vi "set single axis Field Module.vi"(0 "Field Device Select":string(combo)="Elsa Magnet mT", 1 "Field sub select":string(combo)="50mApV", 5 "error in (no error)":errorcluster, 6 "Power dbm":dbl=-135.0 format="%#_13g", 7 "Init":bool, 8 "Field Target mT or dBm":dbl format="%#_13g", 9 "Exec":bool, 10 "Field Rate mT per sec":dbl=0.1 format="%#_13g", 11 "final":bool) -> (19 "error out":errorcluster)   [LabVIEW 2024]
panel:
  out "Voltage controlled Field mT 2":dbl
  in  "E8257 VISA":refnum<visa-resource-name>="GPIB0::19::INSTR"
  out "Current FIeld mT":dbl
  out "Voltage controlled Field mT":dbl
  # "1mT =?V"
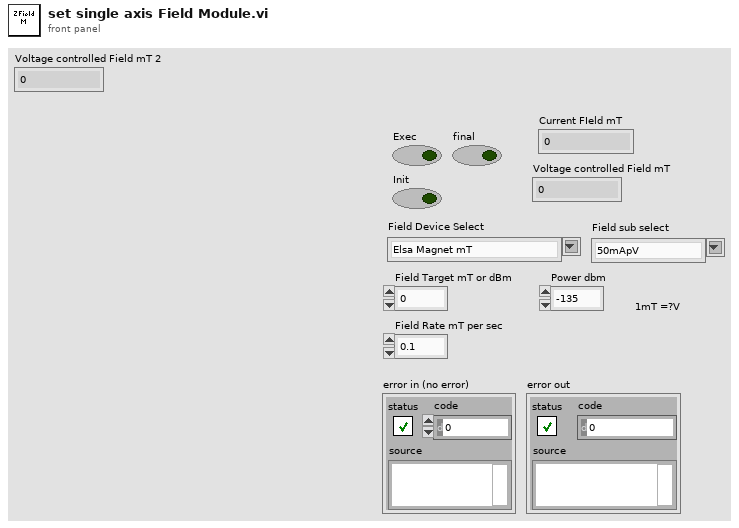
[diagram p1: front panel]
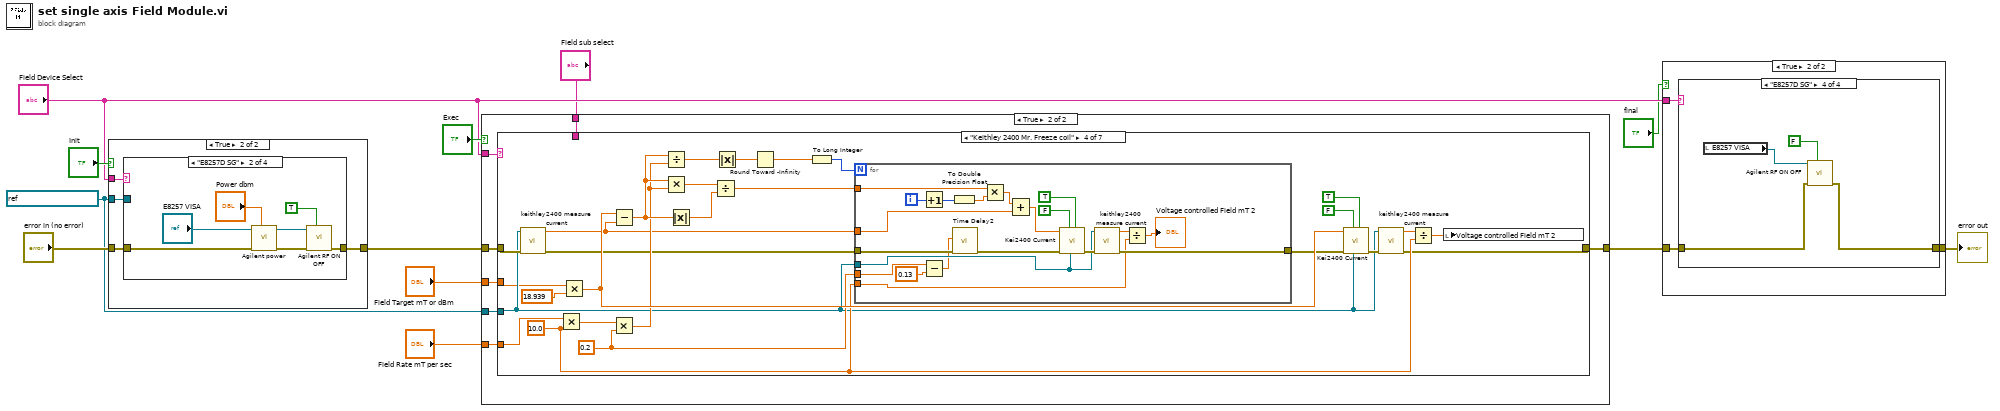
[diagram p0: block diagram]
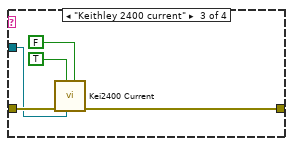
[diagram p8: hidden frame]
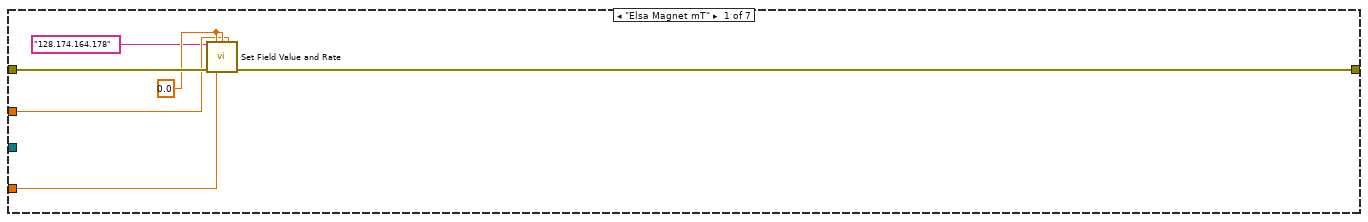
[diagram p11: hidden frame]
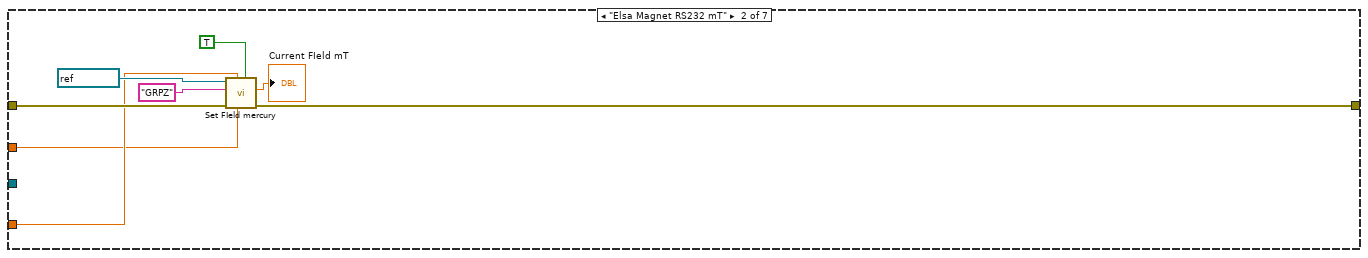
[diagram p12: hidden frame]
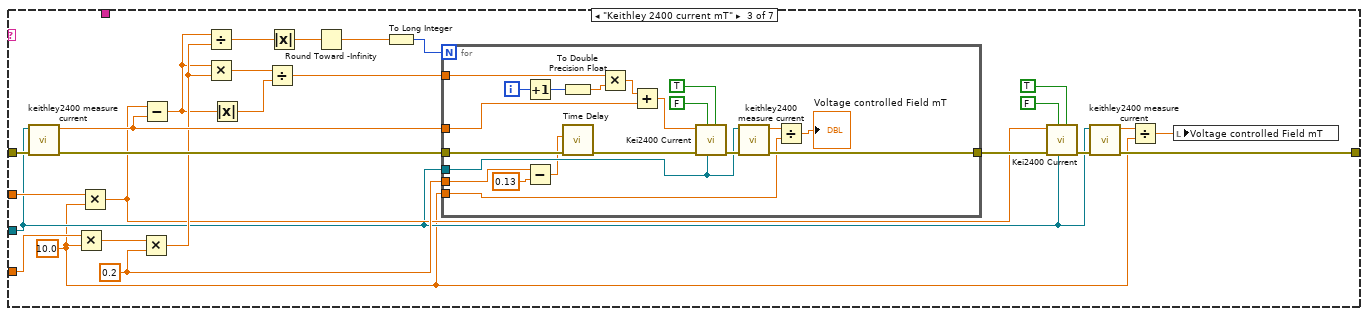
[diagram p13: hidden frame]
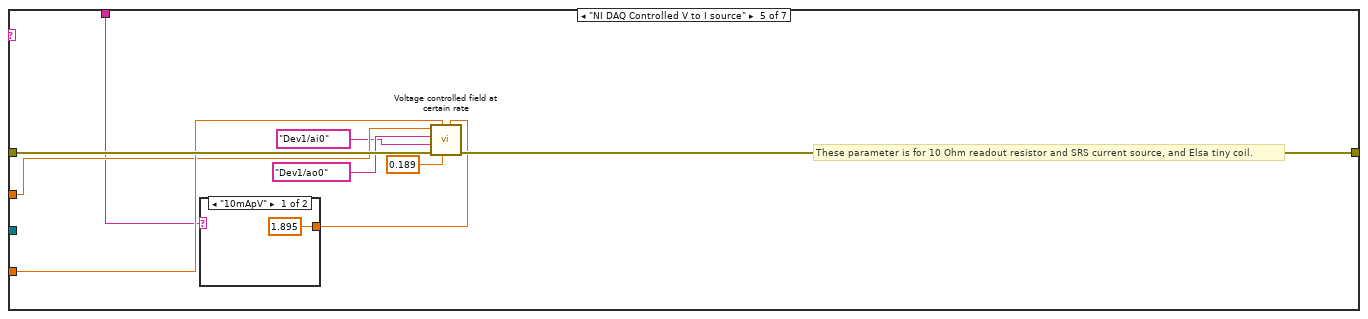
[diagram p14: hidden frame]
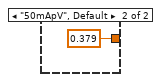
[diagram p15: hidden frame]
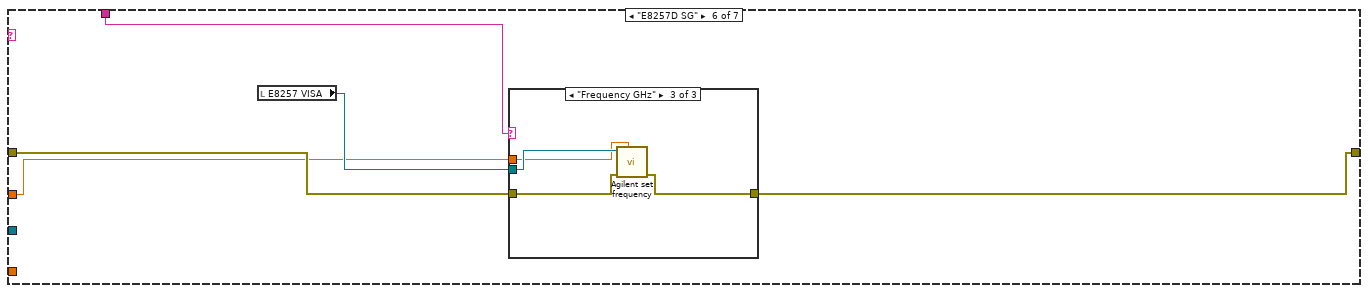
[diagram p16: hidden frame]
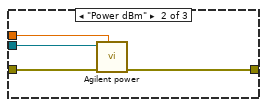
[diagram p18: hidden frame]
diagram:
  w2 = refnum<visa-resource-name> "GPIB0::26::INSTR" ("VISA resource name")
  n1 = case shown="True" "Init" {
    tunnel: "error in (no error)" -> [w13 w17]
    tunnel: [w13 w16] -> w7
    tunnel: "Field Device Select" -> [_ w15]
    tunnel: w2 -> [_ w14]
    frame False {
    }
    frame True {
      n2 = case shown="\"E8257D SG\"" w15 {
        tunnel: w17 -> [w18 w25 w28 w31]
        tunnel: [w18 w19 w27 w31] -> w16
        tunnel: w14 -> [_ _ w26 _]
        frame "Elsa Magnet" {
        }
        frame "E8257D SG" {
          n3 = call "Agilent power.vi"("Power dbm"="Power dbm", "error in (no error)"=w25, "VISA resource name"="E8257 VISA") -> ("error out"=w21:errorcluster, "VISA resource name out"=w22:refnum<visa-resource-name>)  [unwired: 7 in]
          n4 = call "Agilent RF ON OFF.vi"("Output Enable"=TRUE, "error in (no error)"=w21, "VISA resource name"=w22) -> ("error out"=w19:errorcluster)  [unwired: 7 in, 1 out]
        }
        frame "Keithley 2400 current" {
          n5 = call "Kei2400 Current.vi"("Exec"=FALSE, "VISA resource name"=w26, "Init"=TRUE, "error in (no error)"=w28) -> ("error out"=w27:errorcluster)  [unwired: 7 in]
        }
        frame "None", Default {
        }
      }
    }
  }
  n6 = case shown="True" "Exec" {
    tunnel: w7 -> [w32 w39]
    tunnel: [w32 w34] -> w5
    tunnel: "Field Target mT or dBm" -> [_ w38]
    tunnel: "Field Rate mT per sec" -> [_ w37]
    tunnel: "Field Device Select" -> [_ w36]
    tunnel: w2 -> [_ w35]
    tunnel: "Field sub select" -> [_ w33]
    frame False {
    }
    frame True {
      n7 = case shown="\"Keithley 2400 Mr. Freeze coil\"" w36 {
        tunnel: w39 -> [w45 w53 w78 w103 w155 w161 w172]
        tunnel: w38 -> [w42 w48 w79 w101 w153 w159 _]
        tunnel: w37 -> [w41 w49 w77 w104 w154 _ _]
        tunnel: w35 -> [_ _ w57 w102 _ _ _]
        tunnel: [w44 w50 w58 w105 w150 w160 w172] -> w34
        tunnel: w33 -> [_ _ _ _ w147 w158 _]
        frame "Elsa Magnet mT" {
          w43 = 0.0 ("Target Field X kG")
          n8 = call "Set Field Value and Rate.vi"("IP Address"="128.174.164.178", "Target Field X mT"=w43, "Target Field Y mT"=w43, "Target Field Z mT"=w42, "error in (no error)"=w45, "Ramp Rate mT per s"=w41) -> ("error out"=w44:errorcluster)  [unwired: 9 in]
        }
        frame "Elsa Magnet RS232 mT" {
          n9 = call "Set FIeld mercury.vi"("wait for hold"=TRUE, "FIeld mT"=w48, "FIeld mT  per sec"=w49, "error in (no error)"=w53, "Device on PSU"="GRPZ", "VISA resource name"=refnum<visa-resource-name> "COM1") -> ("error out"=w50:errorcluster, "Current FIeld mT"=→"Current FIeld mT":dbl)  [unwired: 3 in, 1 out]
        }
        frame "Keithley 2400 current mT" {
          w72 = 0.2 ("y")
          w54 = 10.0 ("y")
          n10 = call "keithley2400 measure current.vi"("error in (no error)"=w78, "VISA resource name"=w57) -> ("error out"=w75:errorcluster, "Current mA"=w73:dbl)  [unwired: 8 in]
          n11 = Multiply(x=w77, y=w54) -> (x*y=w76:dbl)
          n12 = Multiply(x=w79, y=w54) -> (x*y=w62:dbl)
          n13 = Multiply(x=w76, y=w72) -> (x*y=w71:dbl)
          n14 = Subtract(x=w62, y=w73) -> (x-y=w69:dbl)
          n15 = Divide(x=w69, y=w71) -> (x/y=w74:dbl)
          n16 = Multiply(x=w69, y=w71) -> (x*y=w70:dbl)
          n17 = Absolute Value(x=w69) -> (abs(x)=w68:dbl)
          n18 = Divide(x=w70, y=w68) -> (x/y=w67:dbl)
          n19 = Absolute Value(x=w74) -> (abs(x)=w66:dbl)
          n20 = Round Toward -Infinity(1:w66) -> (0:w65:dbl)
          n21 = To Long Integer(number=w65) -> (32bit integer=w64:i32)
          n22 = for {
            N: w64 -> [_]
            tunnel: w57 -> [w88]
            tunnel: w75 -> [w92]
            tunnel: [w86] -> w63
            tunnel: w73 -> [w93]
            tunnel: w72 -> [w85]
            tunnel: w67 -> [w90]
            tunnel: w54 -> [w80]
            i -> [w97]
            n23 = Increment(x=w97) -> (x+1=w96:i32)
            n24 = Subtract(x=w85, y=0.13) -> (x-y=w83:dbl)
            n25 = To Double Precision Float(number=w96) -> (double precision float=w95:dbl)
            n26 = call "Time Delay"("error in (no error)"=w92, "Delay Time (s)"=w83) -> ("error out"=w87:errorcluster)  [unwired: 9 in]
            n27 = Multiply(x=w90, y=w95) -> (x*y=w94:dbl)
            n28 = Add(x=w94, y=w93) -> (x+y=w91:dbl)
            n29 = call "Kei2400 Current.vi"("Exec"=TRUE, "VISA resource name"=w88, "Init"=FALSE, "error in (no error)"=w87, "Current mA"=w91) -> ("error out"=w89:errorcluster)  [unwired: 6 in]
            n30 = call "keithley2400 measure current.vi"("error in (no error)"=w89, "VISA resource name"=w88) -> ("error out"=w86:errorcluster, "Current mA"=w81:dbl)  [unwired: 8 in]
            n31 = Divide(x=w81, y=w80) -> (x/y=→"Voltage controlled Field mT":dbl)
          }
          n32 = call "Kei2400 Current.vi"("Exec"=TRUE, "VISA resource name"=w57, "Init"=FALSE, "error in (no error)"=w63, "Current mA"=w62) -> ("error out"=w59:errorcluster)  [unwired: 6 in]
          n33 = call "keithley2400 measure current.vi"("error in (no error)"=w59, "VISA resource name"=w57) -> ("error out"=w58:errorcluster, "Current mA"=w55:dbl)  [unwired: 8 in]
          n34 = Divide(x=w55, y=w54) -> (x/y=w56:dbl)
          n35 = local write "Voltage controlled Field mT"(w56) -> ()
        }
        frame "Keithley 2400 Mr. Freeze coil" {
          w108 = 0.2 ("y")
          w109 = 10.0 ("y")
          n36 = call "keithley2400 measure current.vi"("error in (no error)"=w103, "VISA resource name"=w102) -> ("error out"=w111:errorcluster, "Current mA"=w113:dbl)  [unwired: 8 in]
          n37 = Multiply(x=w104, y=w109) -> (x*y=w110:dbl)
          n38 = Multiply(x=w101, y=18.939) -> (x*y=w123:dbl)
          n39 = Multiply(x=w110, y=w108) -> (x*y=w114:dbl)
          n40 = Subtract(x=w123, y=w113) -> (x-y=w116:dbl)
          n41 = Divide(x=w116, y=w114) -> (x/y=w112:dbl)
          n42 = Multiply(x=w116, y=w114) -> (x*y=w115:dbl)
          n43 = Absolute Value(x=w116) -> (abs(x)=w117:dbl)
          n44 = Divide(x=w115, y=w117) -> (x/y=w118:dbl)
          n45 = Absolute Value(x=w112) -> (abs(x)=w119:dbl)
          n46 = Round Toward -Infinity(1:w119) -> (0:w120:dbl)
          n47 = To Long Integer(number=w120) -> (32bit integer=w121:i32)
          n48 = for {
            N: w121 -> [_]
            tunnel: w102 -> [w135]
            tunnel: w111 -> [w139]
            tunnel: [w133] -> w122
            tunnel: w113 -> [w140]
            tunnel: w108 -> [w132]
            tunnel: w118 -> [w137]
            tunnel: w109 -> [w127]
            i -> [w144]
            n49 = Increment(x=w144) -> (x+1=w143:i32)
            n50 = Subtract(x=w132, y=0.13) -> (x-y=w130:dbl)
            n51 = To Double Precision Float(number=w143) -> (double precision float=w142:dbl)
            n52 = call "Time Delay2"("error in (no error)"=w139, "Delay Time (s)"=w130) -> ("error out"=w134:errorcluster)  [unwired: 9 in]
            n53 = Multiply(x=w137, y=w142) -> (x*y=w141:dbl)
            n54 = Add(x=w141, y=w140) -> (x+y=w138:dbl)
            n55 = call "Kei2400 Current.vi"("Exec"=TRUE, "VISA resource name"=w135, "Init"=FALSE, "error in (no error)"=w134, "Current mA"=w138) -> ("error out"=w136:errorcluster)  [unwired: 6 in]
            n56 = call "keithley2400 measure current.vi"("error in (no error)"=w136, "VISA resource name"=w135) -> ("error out"=w133:errorcluster, "Current mA"=w128:dbl)  [unwired: 8 in]
            n57 = Divide(x=w128, y=w127) -> (x/y=→"Voltage controlled Field mT 2":dbl)
          }
          n58 = call "Kei2400 Current.vi"("Exec"=TRUE, "VISA resource name"=w102, "Init"=FALSE, "error in (no error)"=w122, "Current mA"=w123) -> ("error out"=w124:errorcluster)  [unwired: 6 in]
          n59 = call "keithley2400 measure current.vi"("error in (no error)"=w124, "VISA resource name"=w102) -> ("error out"=w105:errorcluster, "Current mA"=w126:dbl)  [unwired: 8 in]
          n60 = Divide(x=w126, y=w109) -> (x/y=w125:dbl)
          n61 = local write "Voltage controlled Field mT 2"(w125) -> ()
        }
        frame "NI DAQ Controlled V to I source" {
          # "These parameter is for 10 Ohm readout resistor and SRS current source, and Elsa tiny coil."
          n62 = case shown="\"10mApV\"" w147 {
            tunnel: [1.895 ("output voltage per mT") 0.379 ("output voltage per mT")] -> w149
            frame "10mApV" {
            }
            frame "50mApV", Default {
            }
          }
          n63 = call "Voltage controlled field at certain rate.vi"("action voltage per mT"=w149, "Readout voltage per mT"=0.189 ("intput voltage per mT"), "Rate mT per sec"=w154, "error in (no error)"=w155, "Voltage read channel"=tag "Dev1/ai0", "Voltage output channel"=tag "Dev1/ao0", "Target field mT"=w153) -> ("error out"=w150:errorcluster)  [unwired: 4 in]
        }
        frame "E8257D SG" {
          n64 = local read "E8257 VISA"() -> (w162:refnum<visa-resource-name>)
          n65 = case shown="\"Frequency GHz\"" w158 {
            tunnel: w162 -> [_ w167 w169]
            tunnel: w161 -> [w163 w166 w171]
            tunnel: [w163 w165 w170] -> w160
            tunnel: w159 -> [_ w164 w168]
            frame "None", Default {
            }
            frame "Power dBm" {
              n66 = call "Agilent power.vi"("Power dbm"=w164, "error in (no error)"=w166, "VISA resource name"=w167) -> ("error out"=w165:errorcluster)  [unwired: 7 in, 1 out]
            }
            frame "Frequency GHz" {
              n67 = call "Agilent set frequency.vi"("Frequency GHz"=w168, "error in (no error)"=w171, "VISA resource name"=w169) -> ("error out"=w170:errorcluster)  [unwired: 7 in, 1 out]
            }
          }
        }
        frame "None", Default {
        }
      }
    }
  }
  n68 = case shown="True" "final" {
    tunnel: w5 -> [w173 w176]
    tunnel: [w173 w175] -> w4
    tunnel: "Field Device Select" -> [_ w174]
    frame False {
    }
    frame True {
      n69 = case shown="\"E8257D SG\"" w174 {
        tunnel: w176 -> [w177 w178 w179 w183]
        tunnel: [w177 w178 w179 w182] -> w175
        frame "Elsa Magnet" {
        }
        frame "Keithley 2400 current" {
        }
        frame "None", Default {
        }
        frame "E8257D SG" {
          n70 = local read "E8257 VISA"() -> (w180:refnum<visa-resource-name>)
          n71 = call "Agilent RF ON OFF.vi"("Output Enable"=FALSE, "error in (no error)"=w183, "VISA resource name"=w180) -> ("error out"=w182:errorcluster)  [unwired: 7 in, 1 out]
        }
      }
    }
  }
  "error out" <- w4
